vi "niRFUtil RFHS Channelizer CreateChannelizerCheckFS CSG.vi"(9 "fs [Hz]":dbl, 11 "error in (no error)":errorcluster) -> (15 "error out":errorcluster)   [LabVIEW 2015, in "niRFUtil.lvlib"]
uses:
  niRFUtil.lvlib
  Includes/niRFUtil RFHS Channelizer ChannelizerErrors.ctl
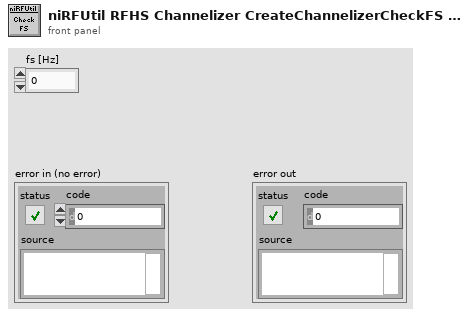
[diagram p1: front panel]
types:
  T1 = typedef "niRFUtil.lvlib/niRFUtil RFHS Channelizer ChannelizerErrors.ctl" = enum32{"No Error", "Invalid Channel", "Internal Error", "Invalid Channel fs", "Invalid Phase Shift", "Invalid fs", "Invalid Number Of Channles", "Invalid FFT Channel fs", "Invalid Resampler Channel fs", "Not a 15kHz Multiple", "Invalid Channel fc", "Invalid passBW/stopBW", "Coerced Rejection", "Requires Internal Buffer", "Duplicated Destination Channel Name", "Configuration Format Error", "Illegal Execution state", "DLL not found", "DLL loading failure", "AVX instruction failure"}
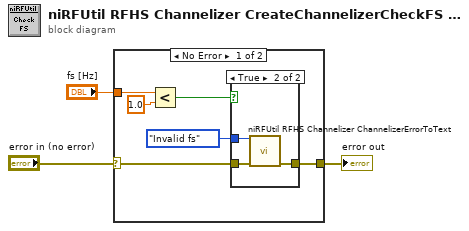
[diagram p0: block diagram]
diagram:
  n1 = case shown="No Error" "error in (no error)" {
    selector: "error in (no error)" -> [w5 w14]
    tunnel: "fs [Hz]" -> [w9 _]
    tunnel: [w4 w14] -> w2
    frame No Error {
      n2 = Less?(x=w9, y=1.0) -> (x < y?=w6:bool)
      n3 = case shown="True" w6 {
        tunnel: w5 -> [w10 w13]
        tunnel: [w10 w12] -> w4
        tunnel: niRFUtil_RFHS_Channelizer_ChannelizerErrors."Invalid fs" ("Error List") -> [_ w11]
        frame False {
        }
        frame True {
          n4 = call "niRFUtil RFHS Channelizer ChannelizerErrorToText.vi"("Error List"=w11, "error in (no error)"=w13) -> ("error out"=w12:errorcluster)  [unwired: 13 in]
        }
      }
    }
    frame Error {
    }
  }
  "error out" <- w2
